vi "EnumArrays.vi"(9 "Array 3":enum32{"a", "b", "c"}[](array[ring]), 10 "Array 2":enum16{"a", "b", "c"}[](array[ring]), 11 "Array 1":enum8{"a", "b", "c"}[](array[ring])) -> ()   [LabVIEW 2014]
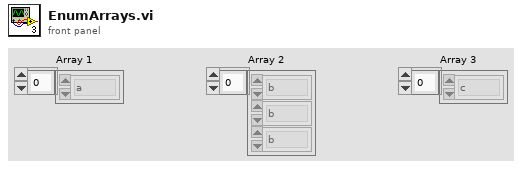
[diagram p1: front panel]
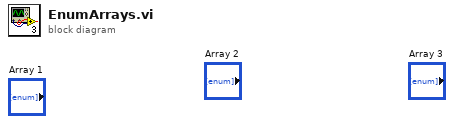
[diagram p0: block diagram]
diagram:
